vi "Profile_Torque_Mode.vi"() -> ()   [LabVIEW 2014]
uses:
  <vilib>/Motion/plugins/Delta SDI Plug-in/Delta Support Files/Test VIs/SDI Status PDOs.ctl
panel:
  in  "1st RxPDO Mapping-TargetTorque":i16
  out "error out":errorcluster
  in  "stop":bool
  out "SDI Status PDOs":T1
  # "6060h:\n\n0: Reserved\n1: Profile Position Mode\n3: Profile Velocity Mode\n4: Profile Torque Mode\n6: Homing Mode\n7: Interpolated Position Mode\n8: Cyclic Synchronous Position Mode\n9: Cyclic Synchronous Velocity Mode\n10: Cyclic Synchronous Torque Mode"
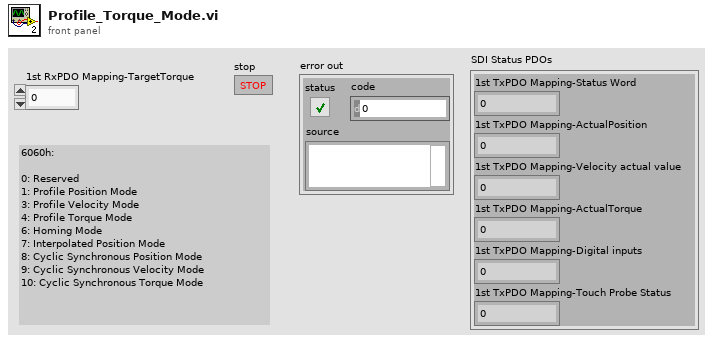
[diagram p1: front panel]
types:
  T1 = typedef "SDI Status PDOs.ctl" = cluster{"1st TxPDO Mapping-Status Word":u16, "1st TxPDO Mapping-ActualPosition":i32, "1st TxPDO Mapping-Velocity actual value":i32, "1st TxPDO Mapping-ActualTorque":i16, "1st TxPDO Mapping-Digital inputs":u32, "1st TxPDO Mapping-Touch Probe Status":u16}
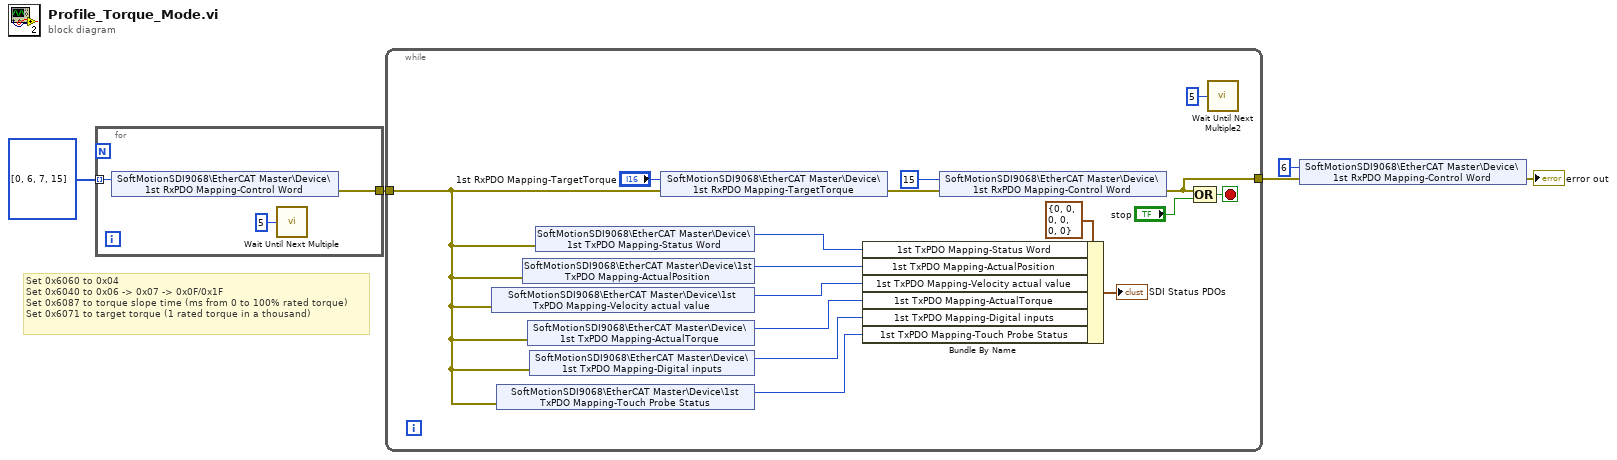
[diagram p0: block diagram]
diagram:
  # "Set 0x6060 to 0x04\nSet 0x6040 to 0x06 -> 0x07 -> 0x0F/0x1F\nSet 0x6087 to torque slope time (ms from 0 to 100% rated torque)\nSet 0x6071 to target torque (1 rated torque in a thousand)"
  n1 = for {
    tunnel: u16[] [0, 6, 7, 15] -> [w8] mode=indexing
    tunnel: [w6] -> w4
    n2 = shared-variable "SoftMotionSDI9068\\EtherCAT Master\\Device\\1st RxPDO Mapping-Control Word"(w8) -> (error out=w6:errorcluster)  [unwired: 1 in]
    n3 = call "Wait Until Next Multiple"("Count(mSec)"=u32 5) -> ()  [unwired: 1 out]
  }
  n4 = while {
    tunnel: w4 -> [w9]
    tunnel: [w10] -> w1
    stop <- w23 stop-if-true
    n5 = shared-variable "SoftMotionSDI9068\\EtherCAT Master\\Device\\1st TxPDO Mapping-Velocity actual value"(error in=w9) -> (w17:i32)  [unwired: 1 out]
    n6 = shared-variable "SoftMotionSDI9068\\EtherCAT Master\\Device\\1st TxPDO Mapping-Touch Probe Status"(error in=w9) -> (w20:u16)  [unwired: 1 out]
    n7 = shared-variable "SoftMotionSDI9068\\EtherCAT Master\\Device\\1st TxPDO Mapping-ActualPosition"(error in=w9) -> (w16:i32)  [unwired: 1 out]
    n8 = shared-variable "SoftMotionSDI9068\\EtherCAT Master\\Device\\1st TxPDO Mapping-ActualTorque"(error in=w9) -> (w18:i16)  [unwired: 1 out]
    n9 = shared-variable "SoftMotionSDI9068\\EtherCAT Master\\Device\\1st TxPDO Mapping-Digital inputs"(error in=w9) -> (w19:u32)  [unwired: 1 out]
    n10 = shared-variable "SoftMotionSDI9068\\EtherCAT Master\\Device\\1st TxPDO Mapping-Status Word"(error in=w9) -> (w15:u16)  [unwired: 1 out]
    n11 = shared-variable "SoftMotionSDI9068\\EtherCAT Master\\Device\\1st RxPDO Mapping-TargetTorque"("1st RxPDO Mapping-TargetTorque", error in=w9) -> (error out=w11:errorcluster)
    n12 = Bundle By Name(cluster=T1 {"1st TxPDO Mapping-Status Word"=0, "1st TxPDO Mapping-ActualPosition"=0, "1st TxPDO Mapping-Velocity actual value"=0, "1st TxPDO Mapping-ActualTorque"=0, "1st TxPDO Mapping-Digital inputs"=0, "1st TxPDO Mapping-Touch Probe Status"=0} ("SDI Status PDOs"), "1st TxPDO Mapping-Status Word"=w15, "1st TxPDO Mapping-ActualPosition"=w16, "1st TxPDO Mapping-Velocity actual value"=w17, "1st TxPDO Mapping-ActualTorque"=w18, "1st TxPDO Mapping-Digital inputs"=w19, "1st TxPDO Mapping-Touch Probe Status"=w20) -> (→"SDI Status PDOs":T1)
    n13 = shared-variable "SoftMotionSDI9068\\EtherCAT Master\\Device\\1st RxPDO Mapping-Control Word"(u16 15 ("1st RxPDO Mapping-Control Word"), error in=w11) -> (error out=w10:errorcluster)
    n14 = Compound Arithmetic op=OR(w10, "stop") -> (w23:bool)
    n15 = call "Wait Until Next Multiple2"("Count(mSec)"=u32 5) -> ()  [unwired: 1 out]
  }
  n16 = shared-variable "SoftMotionSDI9068\\EtherCAT Master\\Device\\1st RxPDO Mapping-Control Word"(u16 6 ("1st RxPDO Mapping-Control Word"), error in=w1) -> (error out=→"error out":errorcluster)
